vi "Test1.vi"() -> ()   [LabVIEW 2020]
panel:
  out "arguments Out":string[](array[string])
  out "application name In":string
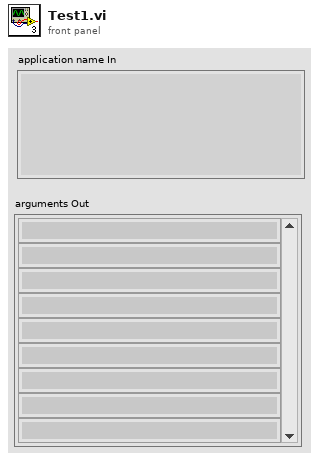
[diagram p1: front panel]
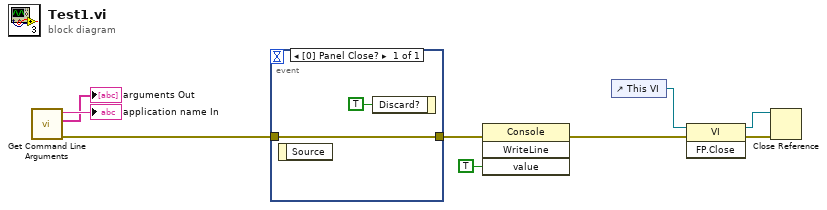
[diagram p0: block diagram]
diagram:
  n1 = call <vilib>:"Get Command Line Arguments.vi"() -> ("error out"=w2:errorcluster, "arguments"=→"arguments Out":string[], "application name"=→"application name In":string)  [unwired: 9 in]
  n2 = event shown="[0] Panel Close?" {
    selector: _ -> [_]
    dyn-events: _ -> [_]
    timeout: _ -> [_]
    tunnel: w2 -> [w11]
    tunnel: [w11] -> w1
    event Panel Close? {
      n3 = event-data() -> ()  [unwired: 1 in, 1 out]
      n4 = event-data("Discard?"=TRUE) -> ()  [unwired: 1 in, 1 out]
    }
  }
  n5 = invoke class="Console" method="WriteLine"(error in=w1, "value"=TRUE) -> (error out=w6:errorcluster)  [unwired: 2 in, 3 out]
  n6 = control-ref of="This VI"() -> (w5:refnum<vi>)
  n7 = invoke class="VI" method="FP.Close"(reference=w5, error in=w6) -> (reference out=w3:refnum<vi>, error out=w4:errorcluster)  [unwired: 1 in, 1 out]
  n8 = Close Reference(reference=w3, error in (no error)=w4) -> ()  [unwired: 1 out]
